vi "System Packed.vi"(8 "error in (no error)":errorcluster) -> (0 "error out":errorcluster, 3 "packed_clusters":bool)   [LabVIEW 2021, in "DataTypes_CIF_U.lvlib"]
doc: "Check if the clusters in Labview are stored as packed structs in memory. If not, padding can be added in between members of a cluster in the device memory."
uses:
  DataTypes_CIF_U.lvlib
  3dc0eadb-47e9-4193-b459-d0fc48cb577a.vi
  3dc0eadb-47e9-4193-b459-d0fc48cb577a.vi/7a63caab-3905-4750-8bef-3ed6d8464949.vi
  3dc0eadb-47e9-4193-b459-d0fc48cb577a.vi/ffc2c926-dd68-4b2a-8345-bf3c85a36d62.vi
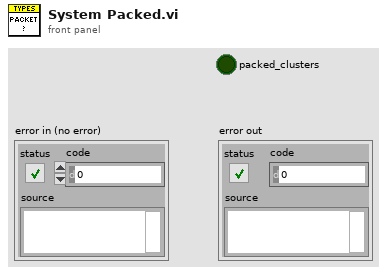
[diagram p1: front panel]
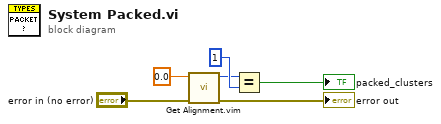
[diagram p0: block diagram]
diagram:
  n1 = call "Get Alignment.vim"("error in (no error)"="error in (no error)", "data"=0.0) -> ("error out"=→"error out":errorcluster, "byte_alignment"=w2:i16)  [unwired: 8 in]
  n2 = Equal?(x=w2, y=i16 1) -> (x = y?=→"packed_clusters":bool)
